vi "Approach then IT VUW.vi"(7 "Computer called (T/F)":bool) -> ()   [LabVIEW 2023]
uses:
  Sub_Vi/TypeDefsControls/Zposition.ctl
  Sub_Vi/TypeDefsControls/Piezo Velocity.ctl
  Sub_Vi/TypeDefsControls/Voltage.ctl
  Sub_Vi/TypeDefsControls/Xposition.ctl
  Sub_Vi/TypeDefsControls/Yposition.ctl
  Sub_Vi/TypeDefsControls/Time.ctl
  Sub_Vi/TypeDefs/WayPointCluster.ctl
  Sub_Vi/TypeDefs/ChangeOnFly.ctl
  Sub_Vi/TypeDefs/Display.ctl
  Sub_Vi/TypeDefs/Settings.ctl
  Sub_Vi/TypeDefsControls/Feedback Type.ctl
  Settings.vi
panel:
  in  "Feedback \nThreshold (A)\nNegative":dbl
  in  "Greater Than 2":bool
  in  "Tab Control 2":T1(tab)
  out "C1":dbl[](graph)
  out "C2":dbl[](graph)
  out "C3":dbl[](graph)
  in  "Feedback Type":T2=enum."Current 1"
  in  "Tab Control":enum32{"C1 vs Z", "C2 vs Z", "C3 vs Z"}(tab)
  out "Z vs C1":cluster{"Y":dbl[], "Y":dbl[]}[](graph)
  out "Z vs C2":cluster{"Y":dbl[], "Y":dbl[]}[](graph)
  out "Z vs C3":cluster{"Y":dbl[], "Y":dbl[]}[](graph)
  in  "SettingsCluster":T3={"Sample Rate (us)"=1, "Samples Per Data Point (int, power of 2)"=1000, "DistanceToBulk (um)"=-1.0, "HoldTimeScaler"=1, "SaveData"=TRUE, "DistanceToBulk (um) 2"=-1.0, "DistanceToBulk (um) 3"=-1.0}
  in  "Display Cluster":T4
  in  "ChangeonFly":T5
  in  "WayPointCluster":T6
  in  "IT Time (s)":T7=8.0 min=0.0
  in  "Start scan Button":bool
  in  "Stop":bool
  in  "Pause":bool
  in  "IT Voltage (V)":T8 min=-10.0 max=10.0
  in  "Greater Than":bool=TRUE
  in  "Set X":bool
  in  "Set Y":bool
  in  "Y":T9=50.0 min=0.0 max=100000.0
  in  "X":T10=50.0 min=0.0 max=100000.0
  in  "Approach Voltage (V)":T8=0.35 min=-10.0 max=10.0
  in  "Approach Rate (µm/s)":T11=0.1 min=0.0
  in  "End Extension (µm)":T12 min=0.0 max=100000.0
  in  "Start Extention (µm)":T12=150.0 min=0.0 max=100000.0
  in  "Feedback \nThreshold (A)\nPositive":dbl
  in  "Start Scanning Button":bool
  out "Lockin Phase":dbl[](graph)
  out "Lockin Amp":dbl[](graph)
  # "Settings"
  # "Pause at"
  # "Advanced Settings"
  # "IT Controls"
  # "Voltage Profile"
  # "Approach"
  # "Retract"
  # "IT"
  # "IT\nVoltage"
  # "Approach\nVoltage"
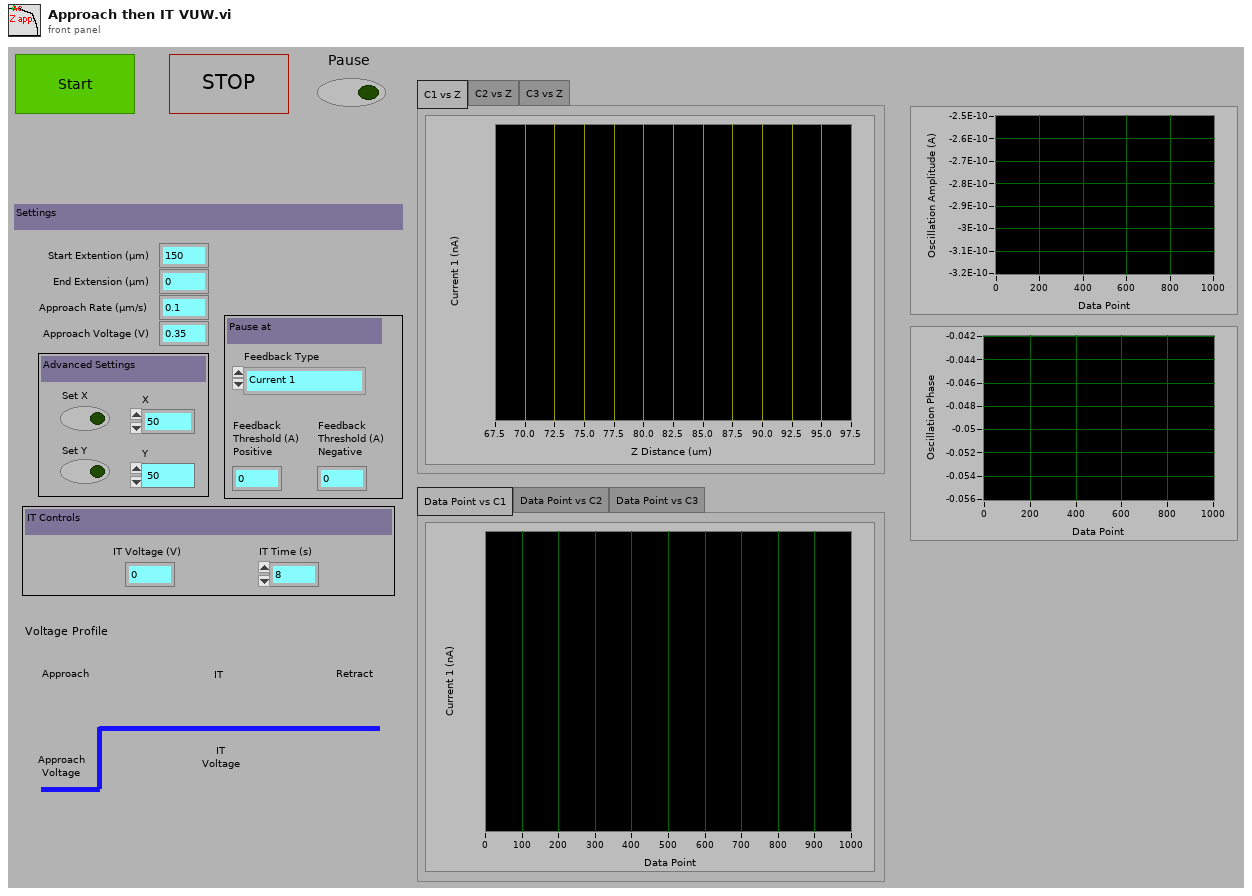
[diagram p1: front panel]
types:
  T1 = enum32{"Data Point vs C1", "Data Point vs C2", "Data Point vs C3"}
  T2 = typedef "Feedback Type.ctl" = enum16{"AC Magnitude", "Current 1", "Current 2", "Phase"}
  T3 = typedef "Settings.ctl" = cluster{"Sample Rate (us)":u32, "Samples Per Data Point (int, power of 2)":i16, "DistanceToBulk (um)":dbl, "HoldTimeScaler":u64, "SaveData":bool, "DistanceToBulk (um) 2":dbl, "DistanceToBulk (um) 3":dbl}
  T4 = typedef "Display.ctl" = cluster{"X":refnum<vi>, "Y":refnum<vi>, "Z":refnum<vi>, "Amp":refnum<vi>, "Phase":refnum<vi>, "t vs Z":refnum<vi>, "t vs C1":refnum<vi>, "t vs C2":refnum<vi>, "t vs C3":refnum<vi>, "t vs Amp":refnum<vi>, "t vs Phase":refnum<vi>, "t vs X":refnum<vi>, "t vs Y":refnum<vi>, "Z vs C1":refnum<vi>, "Z vs C2":refnum<vi>, "Z vs C3":refnum<vi>, "V vs C1":refnum<vi>, "V vs C2":refnum<vi>, "V vs C3":refnum<vi>, "X/Y/Z F":refnum<vi>, "X/Y/Z R":refnum<vi>, "X/Y/C1 F":refnum<vi>, "X/Y/C1 R":refnum<vi>, "X/Y/C2 F":refnum<vi>, "X/Y/C2 R":refnum<vi>, "X/Y/C3 F":refnum<vi>, "X/Y/C3 R":refnum<vi>, "NumberOfLines":u16, "um Per Pixel":dbl, "um Per Line":dbl, "X Center":dbl, "Hop X/Y/Z":refnum<vi>, "Hop X/Y/C1":refnum<vi>, "Hop X/Y/C2":refnum<vi>, "Hop X/Y/C3":refnum<vi>, "X Width":dbl, "Y Width":dbl, "Hopping Distance":dbl, "V2 vs C1":refnum<vi>, "V vs Phase":refnum<vi>, "Y Center":dbl, "Number of Pixels":dbl, "V2 vs C2":refnum<vi>, "V2 vs C3":refnum<vi>, "V vs y":refnum<vi>, "V2 vs y":refnum<vi>, "Z vs Amp":refnum<vi>, "Z vs Phase":refnum<vi>}
  T5 = typedef "ChangeOnFly.ctl" = cluster{"Stop (boolean)":refnum<vi>, "Pause (boolean)":refnum<vi>, "EndCurrentLine (boolean)":refnum<vi>, "max movement per update step (Interger, nm)":refnum<vi>, "P (float, arb)":refnum<vi>, "Feedback set point (double, Amps)":refnum<vi>, "Voltage (double, V)":refnum<vi>, "Feedback set point 2 (double, Amps)":refnum<vi>, "Stop on Greater Than 2? (boolean)":refnum<vi>, "Stop on Greater Than? (boolean)":refnum<vi>, "Voltage 2 (double, V)":refnum<vi>, "Feedback Type (enum)":refnum<vi>, "Feedback Type 2 (enum)":refnum<vi>}
  T6 = typedef "WayPointCluster.ctl" = cluster{"X (um)":dbl[], "Y (um)":dbl[], "Z (um)":dbl[], "V (V)":dbl[], "X Velocity (um s-1)":dbl[], "Y Velocity (um s-1)":dbl[], "Z Velocity (um s-1)":dbl[], "V Velocity (V s-1)":dbl[], "FeedBack Type (enum)":u16[], "Move X (boolean)":bool[], "Move Y (boolean)":bool[], "Move Z (boolean)":bool[], "Move V (boolean)":bool[], "Jump V (boolean)":bool[], "Hold (boolean)":bool[], "Hold Time":u32[], "V2 (V)":dbl[], "Move V2":bool[], "V2 Velocity (V s-1)":dbl[], "Jump V2 (boolean)":bool[], "Update z Position delta (ms)":i16[], "Hold Feedback1":bool[], "Move Z PicoMotor":bool[], " Z PicoMotor Direction":bool[], "DIO0":bool[]}
  T7 = typedef "Time.ctl" = dbl
  T8 = typedef "Voltage.ctl" = dbl
  T9 = typedef "Yposition.ctl" = dbl
  T10 = typedef "Xposition.ctl" = dbl
  T11 = typedef "Piezo Velocity.ctl" = dbl
  T12 = typedef "Zposition.ctl" = dbl
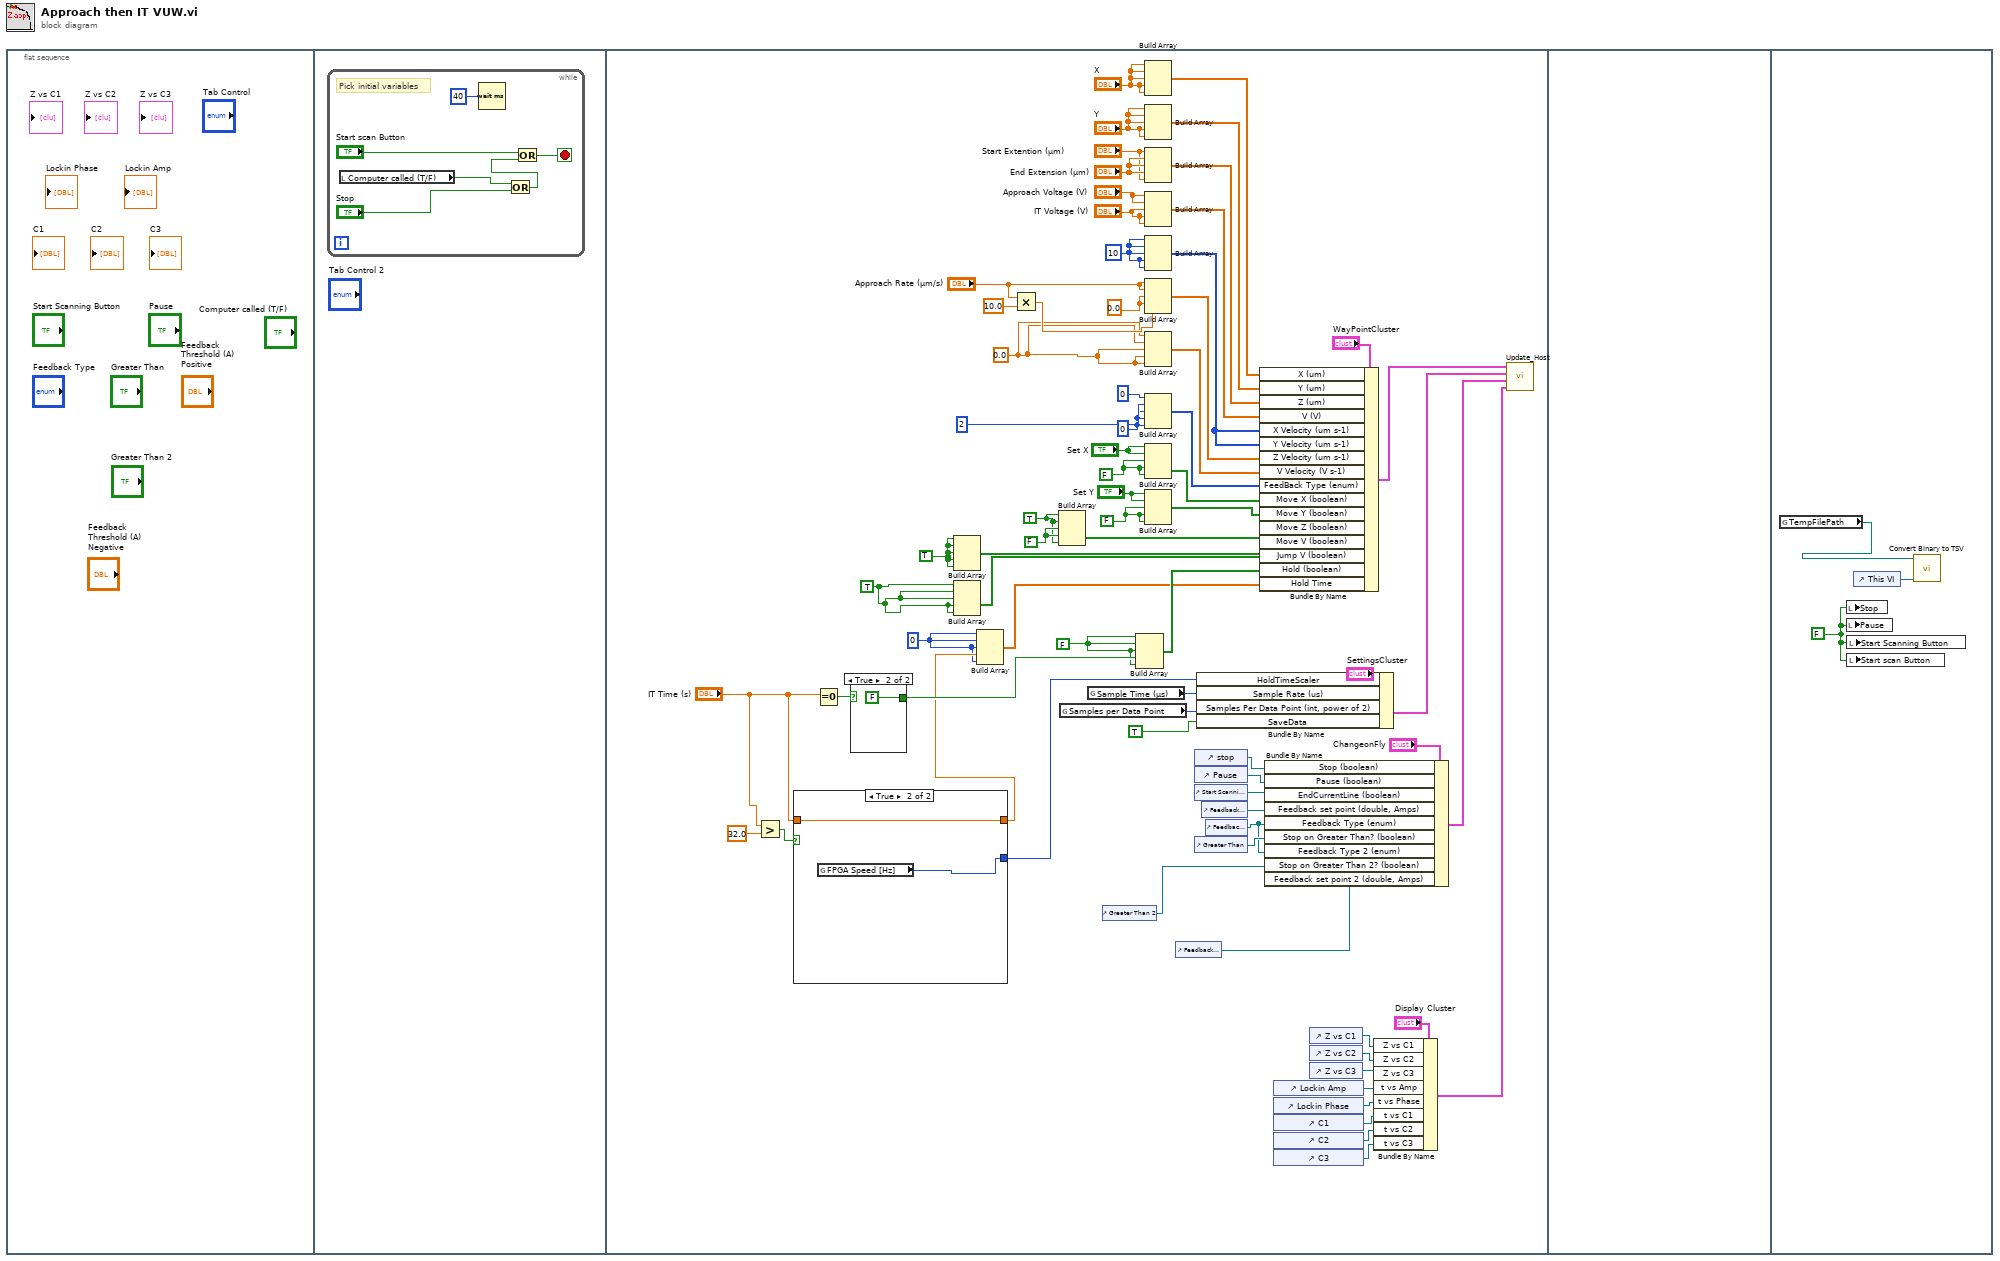
[diagram p0: block diagram]
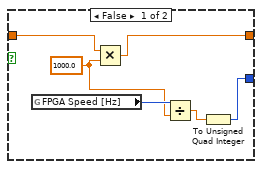
[diagram p2: hidden frame]
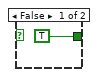
[diagram p3: hidden frame]
diagram:
  n1 = flat-sequence {
    frame #0 {
    }
    frame #1 {
      n2 = while {
        stop <- w6 stop-if-true
        # "Pick initial variables"
        n3 = local read "Computer called (T/F)"() -> (w1:bool)
        n4 = Wait (ms)(milliseconds to wait=u32 40) -> ()  [unwired: 1 out]
        n5 = Or(x=w1, y="Stop") -> (x .or. y?=w2:bool)
        n6 = Or(x="Start scan Button", y=w2) -> (x .or. y?=w6:bool)
      }
    }
    frame #2 {
      w10 = u32 0 ("element")
      w12 = TRUE ("Set Z")
      w13 = TRUE ("element")
      w62 = FALSE ("element")
      w16 = FALSE ("element")
      w15 = FALSE ("element")
      w17 = u16 0 ("element")
      w18 = 0.0
      w41 = 0.0 ("element")
      w11 = FALSE ("Set Z")
      w14 = TRUE ("Set Z")
      w22 = 10
      n7 = Greater?(x="IT Time (s)", y=T7 32.0) -> (0:w31:bool)
      n8 = case shown="True" w31 {
        tunnel: "IT Time (s)" -> [w86 w88]
        tunnel: [w85 w88] -> w29
        tunnel: [w81 w87] -> w28
        frame False {
          w83 = 1000.0 ("y")
          n9 = global read "Settings.vi" "FPGA Speed [Hz]"() -> (w84:i64)
          n10 = Multiply(x=w86, y=w83) -> (x*y=w85:T7)
          n11 = Divide(x=w84, y=w83) -> (x/y=w82:dbl)
          n12 = To Unsigned Quad Integer(1:w82) -> (0:w81:u64)
        }
        frame True {
          n13 = global read "Settings.vi" "FPGA Speed [Hz]"() -> (w87:i64)
        }
      }
      n14 = Equal To 0?(x="IT Time (s)") -> (x = 0?=w61:bool)
      n15 = case shown="True" w61 {
        tunnel: [TRUE ("Set Z") FALSE ("Set Z")] -> w33
        frame False {
        }
        frame True {
        }
      }
      n16 = Build Array(w13, w13, w13, w13, w13) -> (w36:bool[])
      n17 = Build Array(w12, w12, w12, w12, w12) -> (w71:bool[])
      n18 = Build Array(w10, w10, w10, w29, w10) -> (w70:T7[])
      n19 = Multiply(x="Approach Rate (µm/s)", y=T11 10.0) -> (x*y=w19:T11)
      n20 = Build Array(w14, w14, w62, w62, w14) -> (w63:bool[])
      n21 = global read "Settings.vi" "Samples per Data Point"() -> (w66:u16)
      n22 = global read "Settings.vi" "Sample Time (µs)"() -> (w67:u32)
      n23 = control-ref of="Greater Than 2"() -> (w8:refnum<vi>)
      n24 = Build Array(w11, w11, w11, w33, w11) -> (w74:bool[])
      n25 = Build Array("X", "X", "X", "X", "X") -> (w79:T10[])
      n26 = Build Array("Y", "Y", "Y", "Y", "Y") -> (w78:T9[])
      n27 = Build Array("Start Extention (µm)", "End Extension (µm)", "End Extension (µm)", "End Extension (µm)", "Start Extention (µm)") -> (w34:T12[])
      n28 = Build Array("Approach Voltage (V)", "Approach Voltage (V)", "IT Voltage (V)", "IT Voltage (V)", "IT Voltage (V)") -> (w64:T8[])
      n29 = Build Array(w22, w22, w22, w22, w22) -> (w80:i32[])
      n30 = Build Array("Approach Rate (µm/s)", "Approach Rate (µm/s)", w41, w41, w19) -> (w77:T11[])
      n31 = Build Array(w18, w18, w18, w18, w18) -> (w73:dbl[])
      n32 = Build Array(u16 0 ("element"), u16 2, w17, w17, w17) -> (w72:u16[])
      n33 = Build Array("Set X", "Set X", w16, w16, w16) -> (w76:bool[])
      n34 = Build Array("Set Y", "Set Y", w15, w15, w15) -> (w35:bool[])
      n35 = control-ref of="Feedback \nThreshold (A)\nNegative"() -> (w7:refnum<vi>)
      n36 = control-ref of="stop"() -> (w46:refnum<vi>)
      n37 = control-ref of="Pause"() -> (w47:refnum<vi>)
      n38 = control-ref of="Start Scanning Button"() -> (w48:refnum<vi>)
      n39 = control-ref of="Greater Than"() -> (w49:refnum<vi>)
      n40 = Bundle By Name(cluster="SettingsCluster", "HoldTimeScaler"=w28, "Sample Rate (us)"=w67, "Samples Per Data Point (int, power of 2)"=w66, "SaveData"=TRUE) -> (w75:T3)
      n41 = control-ref of="Feedback \nThreshold (A)\nPositive"() -> (w50:refnum<vi>)
      n42 = control-ref of="Feedback Type"() -> (w9:refnum<vi>)
      n43 = Bundle By Name(cluster="WayPointCluster", "X (um)"=w79, "Y (um)"=w78, "Z (um)"=w34, "V (V)"=w64, "X Velocity (um s-1)"=w80, "Y Velocity (um s-1)"=w80, "Z Velocity (um s-1)"=w77, "V Velocity (V s-1)"=w73, "FeedBack Type (enum)"=w72, "Move X (boolean)"=w76, "Move Y (boolean)"=w35, "Move Z (boolean)"=w63, "Move V (boolean)"=w36, "Jump V (boolean)"=w71, "Hold (boolean)"=w74, "Hold Time"=w70) -> (w44:T6)
      n44 = Bundle By Name(cluster="ChangeonFly", "Stop (boolean)"=w46, "Pause (boolean)"=w47, "EndCurrentLine (boolean)"=w48, "Feedback set point (double, Amps)"=w50, "Feedback Type (enum)"=w9, "Stop on Greater Than? (boolean)"=w49, "Feedback Type 2 (enum)"=w9, "Stop on Greater Than 2? (boolean)"=w8, "Feedback set point 2 (double, Amps)"=w7) -> (w51:T5)
      n45 = control-ref of="Lockin Amp"() -> (w59:refnum<vi>)
      n46 = control-ref of="Lockin Phase"() -> (w58:refnum<vi>)
      n47 = control-ref of="C1"() -> (w55:refnum<vi>)
      n48 = control-ref of="C2"() -> (w54:refnum<vi>)
      n49 = control-ref of="C3"() -> (w53:refnum<vi>)
      n50 = control-ref of="Z vs C1"() -> (w69:refnum<vi>)
      n51 = control-ref of="Z vs C2"() -> (w57:refnum<vi>)
      n52 = control-ref of="Z vs C3"() -> (w56:refnum<vi>)
      n53 = Bundle By Name(cluster="Display Cluster", "Z vs C1"=w69, "Z vs C2"=w57, "Z vs C3"=w56, "t vs Amp"=w59, "t vs Phase"=w58, "t vs C1"=w55, "t vs C2"=w54, "t vs C3"=w53) -> (w43:T4)
      n54 = call "Update_Host.vi"("Display Cluster"=w43, "ChangeonFly"=w51, "SettingsCluster"=w75, "WayPointCluster"=w44) -> ()  [unwired: 6 in]
    }
    frame #3 {
    }
    frame #4 {
      w92 = FALSE ("stop recording")
      n55 = global read "Settings.vi" "TempFilePath"() -> (w91:path)
      n56 = local write "Stop"(w92) -> ()
      n57 = local write "Pause"(w92) -> ()
      n58 = local write "Start Scanning Button"(w92) -> ()
      n59 = local write "Start scan Button"(w92) -> ()
      n60 = control-ref of="This VI"() -> (w93:refnum<vi>)
      n61 = call "Convert Binary to TSV.vi"("This VI"=w93, "TDMS DataFile Name"=w91) -> ()  [unwired: 10 in]
    }
  }
